vi "1A Interpret NMEA Sentence.vi"(11 "NMEA Sentence":string) -> ()   [LabVIEW 2011]
doc: "Interprets the NMEA 0813 sentences that we are using from our Airmar PB200 WeatherStation sensor.\nBy Jaime McCandless\nTODO: finish implementing NMEA sentences"
uses:
  2-Think/2 Typedefs/UTM Location.ctl
  2-Think/2 Typedefs/heading.ctl
  2-Think/2 Typedefs/Velocity.ctl
  2-Think/2 Typedefs/apparent wind.ctl
  2-Think/2 Typedefs/pitch and roll.ctl
  2-Think/2 Globals/2 Global.vi
  <vilib>/regexp/Match Regular Expression.xnode
panel:
  out "Defiltering Wind Data":bool=TRUE
  in  "UTC Time Zone":i32=-5
  in  "Tab Control":T1(tab)
  out "GPS (GGA) Data":T2
  out "GPS (GLL) Data":T3
  out "GPGSA Data":T4
  out "UTC Time":timestamp
  out "Local Time":timestamp
  out "Lattitude (ddmm.mmmm)":dbl format="%_8g"
  out "Lattitude North/South":string
  out "Longitude (ddmm.mmmm)":dbl format="%_8g"
  out "Longitude East/West":string
  out "Speed over ground (knots)":dbl format="%_3g"
  out "Course over ground (degrees)":dbl format="%_4g"
  out "Magnetic Variation (degrees)":dbl format="%_4g"
  out "Variation East/West":string
  out "GPS (RMC) Data":T5 {"Course over ground (degrees)" format="%#.6g"; "Speed over ground (knots)" format="%#.6g"; "Magnetic Variation (degrees)" format="%#.6g"; "Longitude (ddmm.mmmm)" format="%#.6g"; "Lattitude (ddmm.mmmm)" format="%#.6g"}
  out "GPS Data Valid?":bool
  out "Robot UTM Location":T6 {"North" format="%#_10f"; "East" format="%#_8f"}
  out "GPS (VTG) Data":T7
  out "Heading":dbl
  out "Turn (ROT) Data":T8
  out "Meteorological Data":T9
  out "Theoretical true wind direction":T10(graph)
  out "Relative wind direction":cluster{dbl, "Filtered Value Out":dbl}(graph)
  out "Wind (MWV) Data, Theoretical":T11
  out "Wind (MWV) Data, Relative":T11
  out "Transducer (XDR) B Data":cluster{"Pitch (deg)":dbl, "Roll (deg)":dbl}
  out "Transducer (XDR) A Data":T12
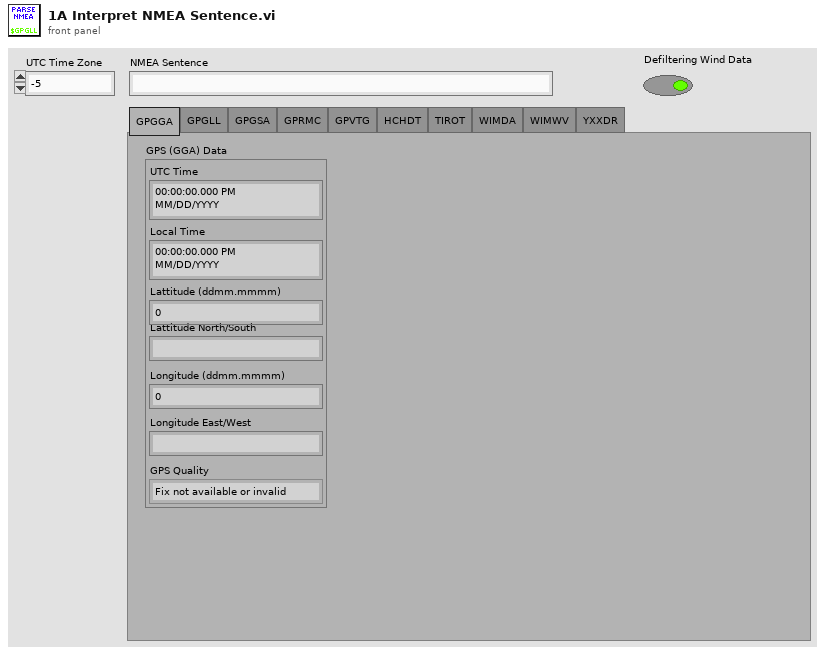
[diagram p1: front panel]
types:
  T1 = enum32{"GPGGA", "GPGLL", "GPGSA", "GPRMC", "GPVTG", "HCHDT", "TIROT", "WIMDA", "WIMWV", "YXXDR"}
  T2 = cluster{"UTC Time":timestamp, "Local Time":timestamp, "Lattitude (ddmm.mmmm)":dbl, "Lattitude North/South":string, "Longitude (ddmm.mmmm)":dbl, "Longitude East/West":string, "GPS Quality":enum16{"Fix not available or invalid", "GPS SPS Mode, fix valid", "Differential GPS, SPS Mode, fix valid", "GPS PPS Mode, fix valid", "Real Time Kinematic (RTK)", "Float RTK", "Estimated (dead reckoning) Mode", "Manual Input Mode", "Simulator Mode"}}
  T3 = cluster{"UTC Time":timestamp, "Local Time":timestamp, "Lattitude (ddmm.mmmm)":dbl, "Lattitude North/South":string, "Longitude (ddmm.mmmm)":dbl, "Longitude East/West":string, "GPS Mode":string, "GPS Data Valid?":bool}
  T4 = cluster{"Mode":string, "Fix Strength":i32, "Satellite IDs":i32[], "PDOP":dbl, "HDOP":dbl, "VDOP":dbl}
  T5 = cluster{"UTC Time":timestamp, "Local Time":timestamp, "Lattitude (ddmm.mmmm)":dbl, "Lattitude North/South":string, "Longitude (ddmm.mmmm)":dbl, "Longitude East/West":string, "Magnetic Variation (degrees)":dbl, "Variation East/West":string, "Speed over ground (knots)":dbl, "Course over ground (degrees)":dbl}
  T6 = typedef "UTM Location.ctl" = cluster{"UTM Zone":dbl, "Hemisphere":enum16{"North", "South"}, "East":dbl, "North":dbl}
  T7 = cluster{"Course Over Ground (True)":dbl, "Course Over Ground (Magnetic)":dbl, "Speed Over Ground (Knots)":dbl, "Speed Over Ground (km/hr)":dbl, "GPS Mode":string}
  T8 = cluster{"Rate of Turn (deg/min)":dbl, "Turn Rotation Data Valid?":bool}
  T9 = cluster{"Barometric Pressure (inches of mercury)":dbl, "Barometric Pressure (bars)":dbl, "Air temperature (degC)":dbl, "Relative humidity (%)":dbl, "Wind direction, True (deg)":dbl, "Wind direction, Magnetic (deg)":dbl, "Wind speed (knots)":dbl, "Wind speed (m/s)":dbl}
  T10 = cluster{"Robot\nHeading ":dbl, "Robot\nHeading ":dbl}
  T11 = cluster{"Angle relative to boat (deg)":dbl, "Wind Data Valid?":bool, "Wind speed (knots)":dbl, "True (T) or Relative (R)":string}
  T12 = cluster{"Calc. Relative Wind Chill (degC)":dbl, "Calc. Theoretical Wind Chill (degC)":dbl, "Calc. Heat Index (degC)":dbl, "Meas. Barometric Pressure (bars)":dbl}
  T13 = cluster{"second":i32, "minute":i32, "hour":i32, "day of month":i32, "month":i32, "year":i32, "day of week":i32, "day of year":i32, "is DST":i32}
  T14 = typedef "heading.ctl" = dbl
  T15 = typedef "Velocity.ctl" = cluster{"East":dbl, "North":dbl}
  T16 = typedef "apparent wind.ctl" = cluster{"Toward Fore":dbl, "Toward Starboard":dbl}
  T17 = typedef "pitch and roll.ctl" = cluster{"Pitch":dbl, "Roll":dbl}
  T18 = typedef "generalized sensor status.ctl" = cluster{"Sensor Connected":T19, "Sensor Initialized":T19, "Sensor OK":T19, "Latest Error String":string, "GPS Lock":T19}
  T19 = typedef "indicator LED.ctl" = bool
  T20 = cluster{"Robot\nHeading ":T14, "Robot\nHeading ":T14}
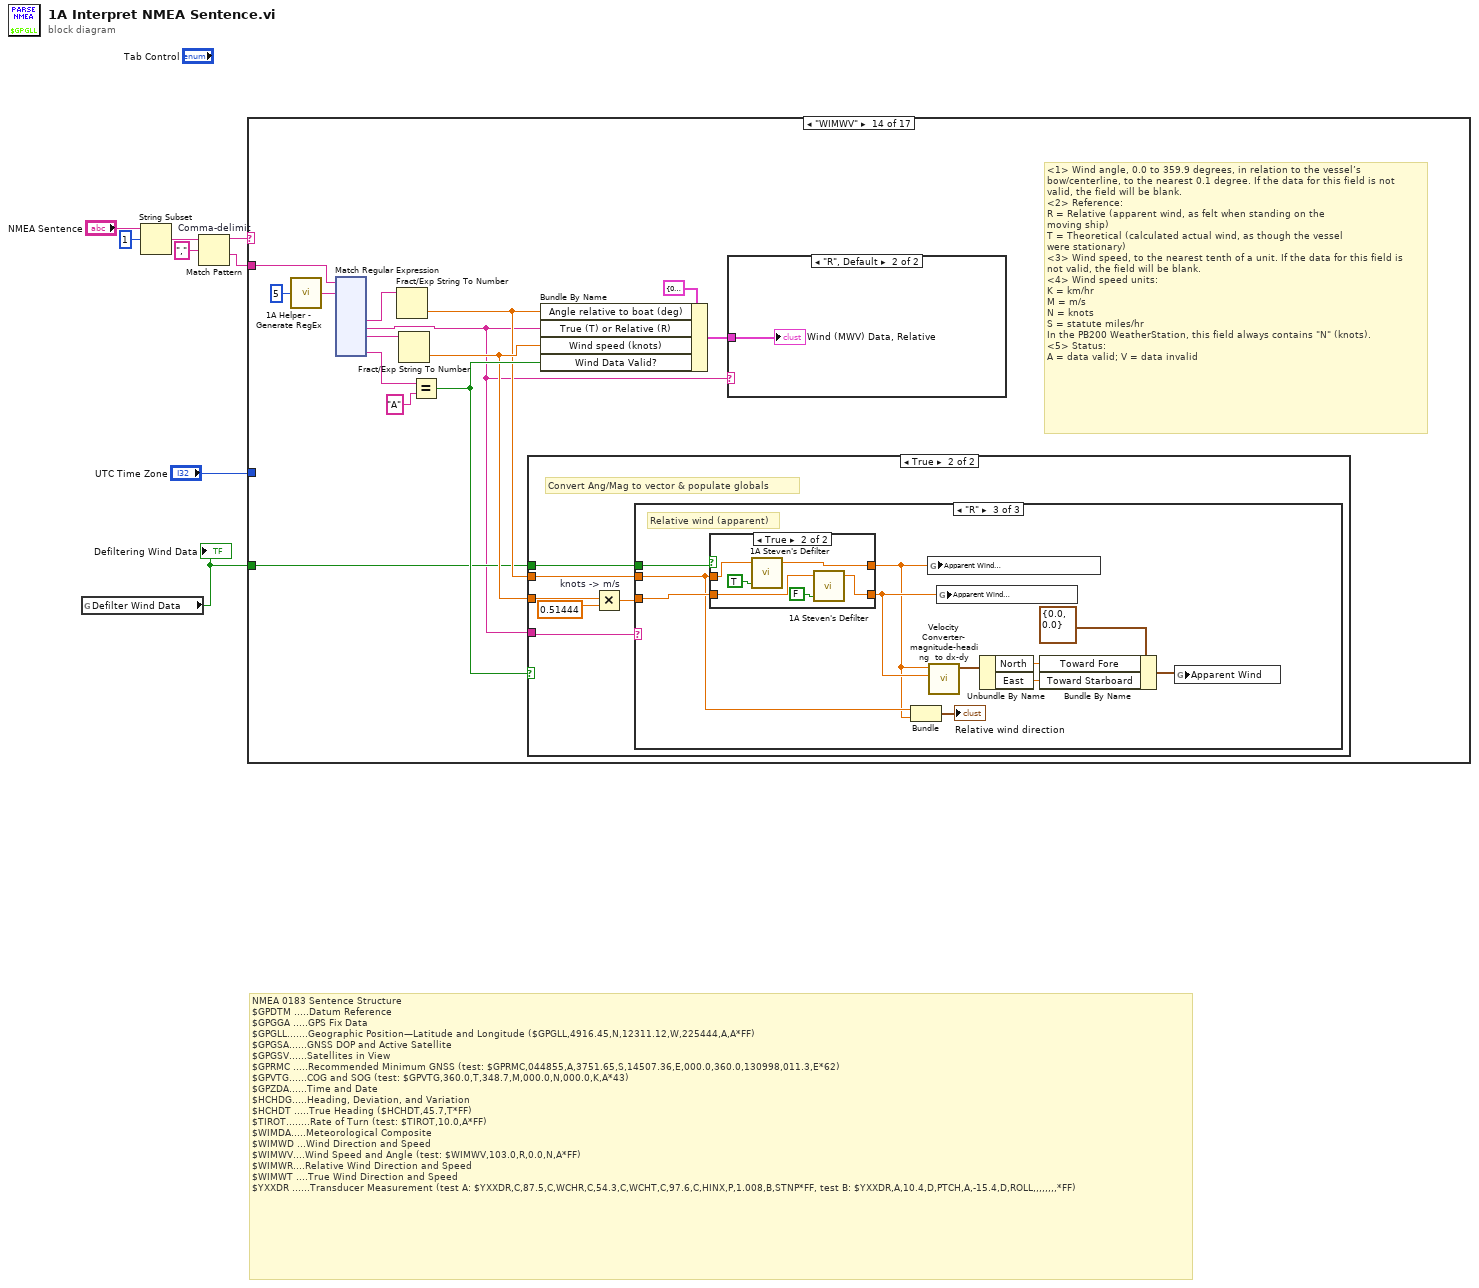
[diagram p0: block diagram]
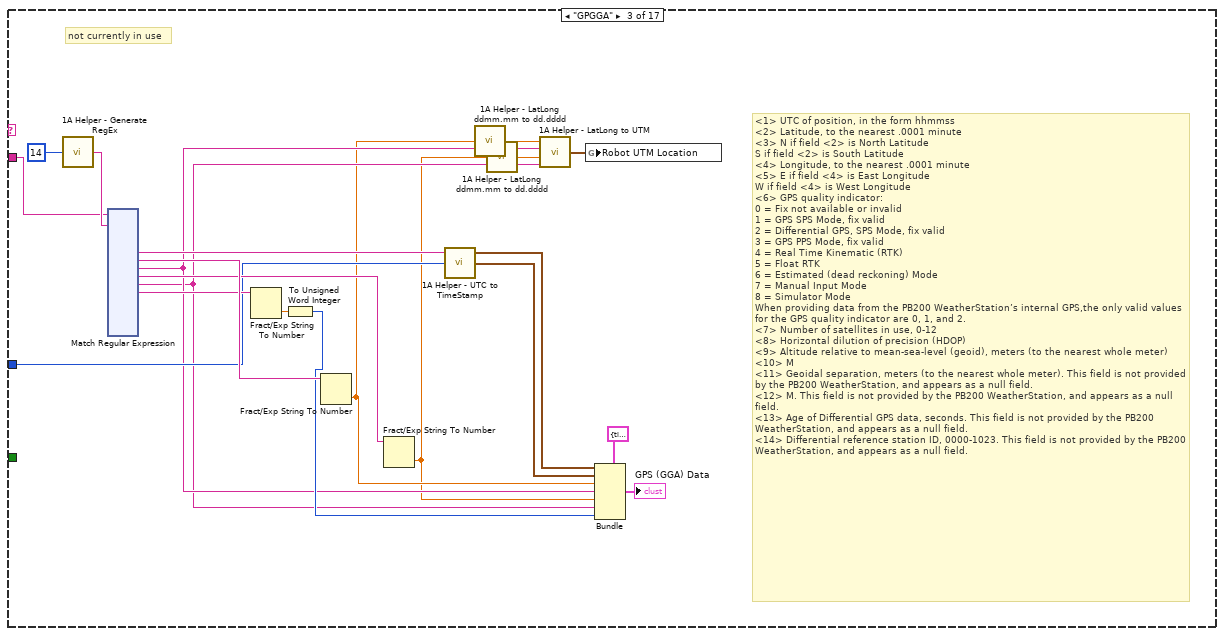
[diagram p4: hidden frame]
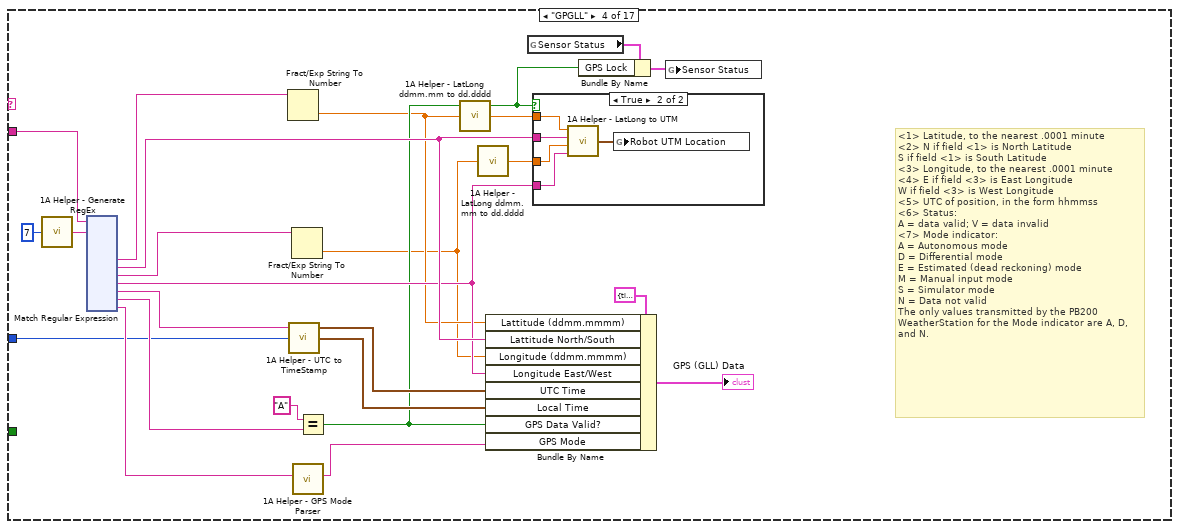
[diagram p5: hidden frame]
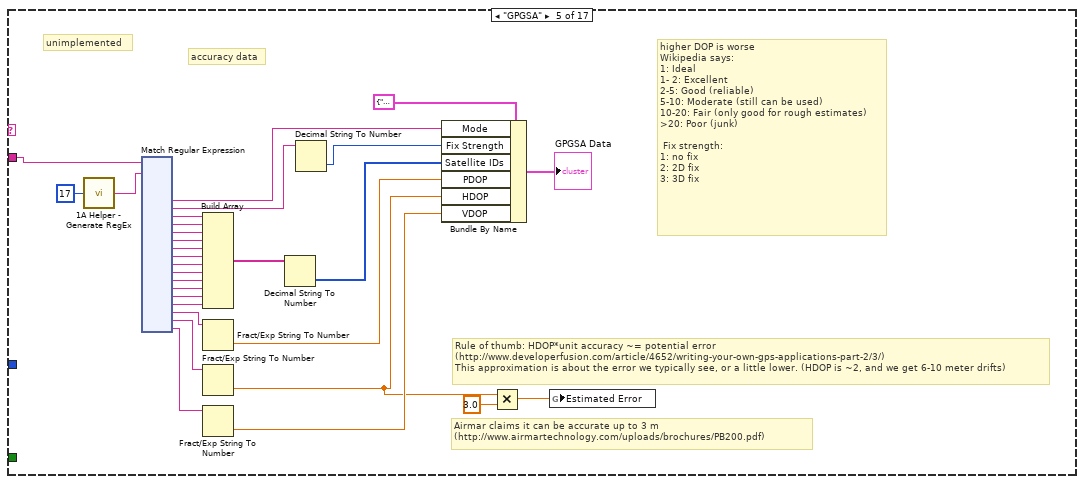
[diagram p7: hidden frame]
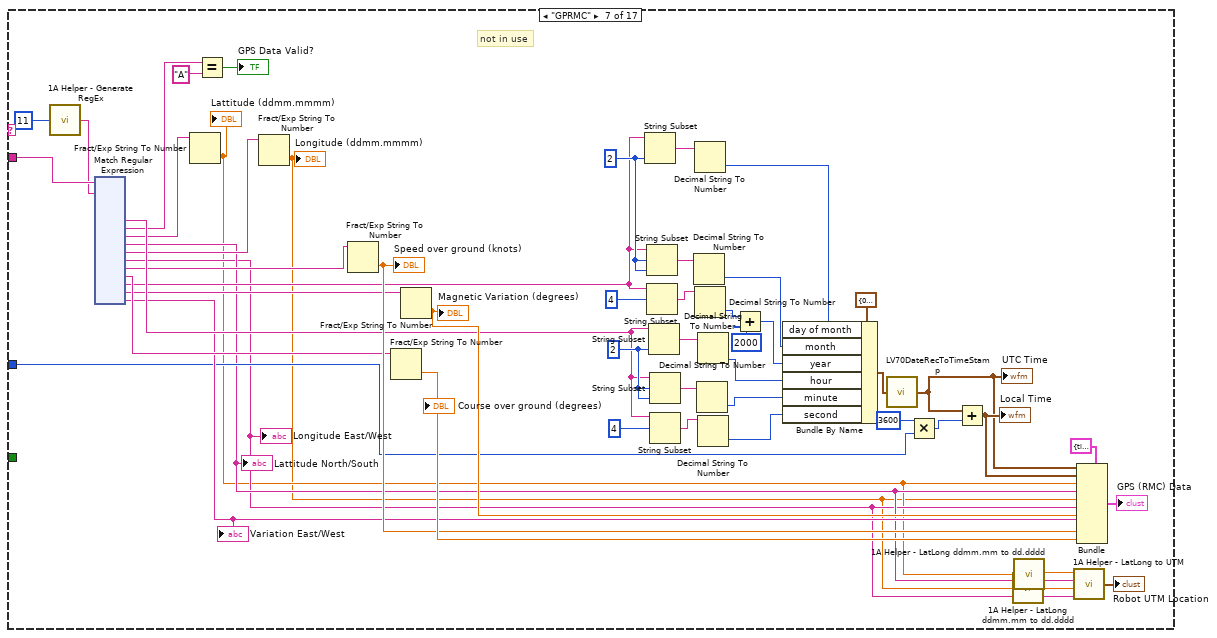
[diagram p9: hidden frame]
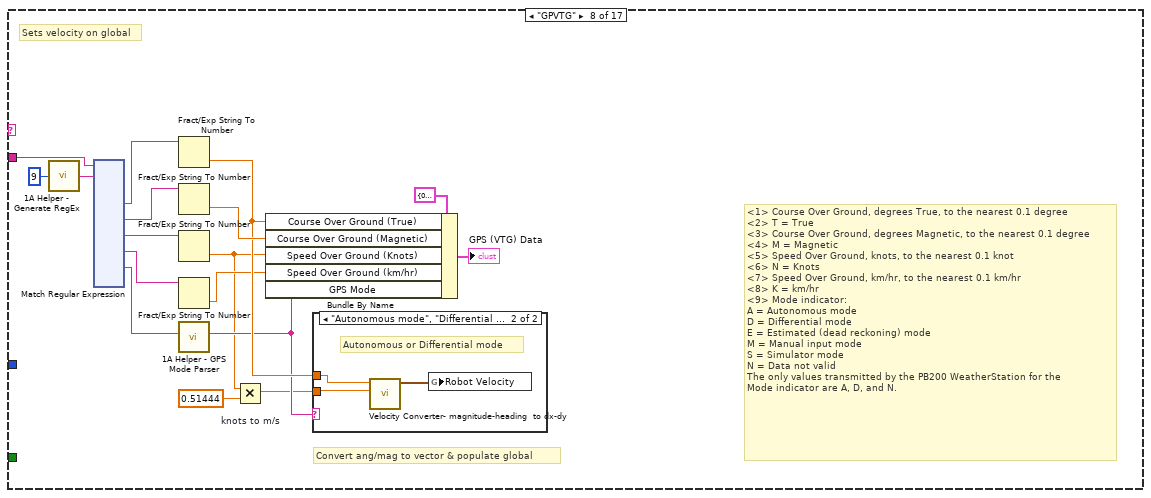
[diagram p10: hidden frame]
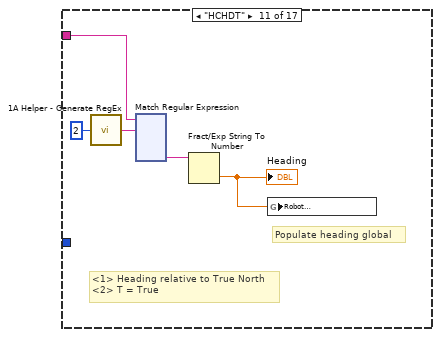
[diagram p14: hidden frame]
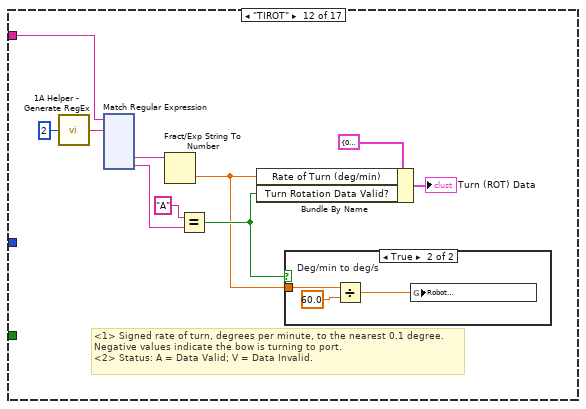
[diagram p15: hidden frame]
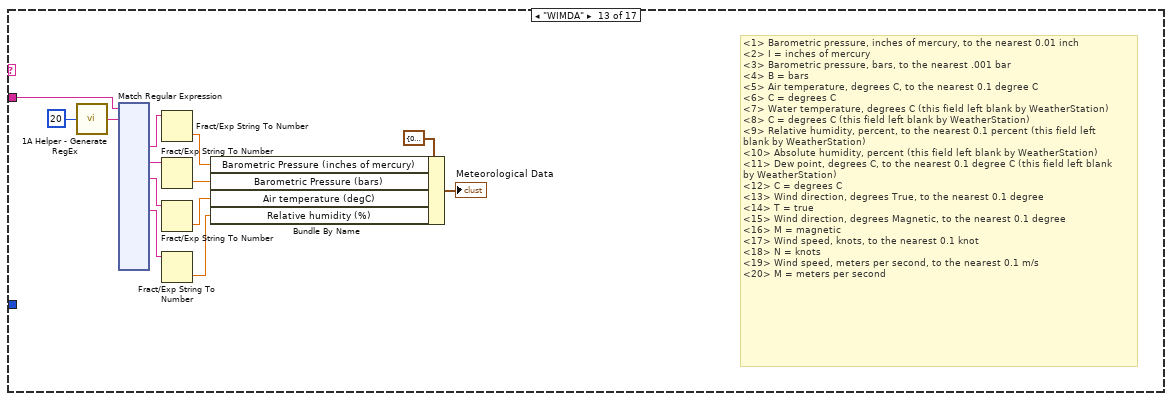
[diagram p17: hidden frame]
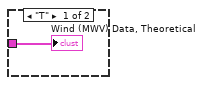
[diagram p18: hidden frame]
diagram:
  # "NMEA 0183 Sentence Structure\n$GPDTM .....Datum Reference\n$GPGGA .....GPS Fix Data\n$GPGLL.......Geographic Position—Latitude and Longitude ($GPGLL,4916.45,N,12311.12,W,225444,A,A*FF)\n$GPGSA......GNSS DOP and Active Satellite\n$GPGSV......Satellites in View\n$GPRMC .....Recommended Minimum GNSS (test: $GPRMC,044855,A,3751.65,S,14507.36,E,000.0,360.0,130998,011.3,E*62)\n$GPVTG......COG and SOG (test: $GPVTG,360.0,T,348.7,M,000.0,N,000.0,K,A*43)\n$GPZDA......Time and Date\n$HCHDG.....Heading, Deviation, and Variation\n$HCHDT .....True Heading ($HCHDT,45.7,T*FF)\n$TIROT........Rate of Turn (test: $TIROT,10.0,A*FF)\n$WIMDA.....Meteorological Composite\n$WIMWD ...Wind Direction and Speed\n$WIMWV....Wind Speed and Angle (test: $WIMWV,103.0,R,0.0,N,A*FF)\n$WIMWR....Relative Wind Direction and Speed\n$WIMWT ....True Wind Direction and Speed\n$YXXDR ......Transducer Measurement (test A: $YXXDR,C,87.5,C,WCHR,C,54.3,C,WCHT,C,97.6,C,HINX,P,1.008,B,STNP*FF, test B: $YXXDR,A,10.4,D,PTCH,A,-15.4,D,ROLL,,,,,,,,*FF)"
  n1 = global read "2 Global.vi" "Defilter Wind Data"() -> (w1:bool)
  "Defiltering Wind Data" <- w1
  n2 = String Subset(string="NMEA Sentence", offset (0)=1) -> (substring=w5:string)  [unwired: 1 in]
  n3 = Match Pattern "Comma-delimit"(string=w5, regular expression=",") -> (before substring=w6:string, after substring=w7:string)  [unwired: 1 in, 2 out]
  n4 = case shown="\"WIMWV\"" w6 {
    tunnel: w7 -> [_ _ w27 w171 w330 _ w479 w648 _ _ w779 w901 w1032 w1172 _ _ w1344]
    tunnel: "UTC Time Zone" -> [_ _ w16 w163 _ _ w467 _ _ _ _ _ _ _ _ _ _]
    tunnel: w1 -> [_ _ _ _ _ _ _ _ _ _ _ _ _ w1164 _ _ _]
    frame "", Default {
    }
    frame "GPDTM" {
      # "unimplemented"
    }
    frame "GPGGA" {
      # "not currently in use"
      # "<1> UTC of position, in the form hhmmss\n<2> Latitude, to the nearest .0001 minute\n<3> N if field <2> is North Latitude\nS if field <2> is South Latitude\n<4> Longitude, to the nearest .0001 minute\n<5> E if field <4> is East Longitude\nW if field <4> is West Longitude\n<6> GPS quality indicator:\n0 = Fix not available or invalid\n1 = GPS SPS Mode, fix valid\n2 = Differential GPS, SPS Mode, fix valid\n3 = GPS PPS Mode, fix valid\n4 = Real Time Kinematic (RTK)\n5 = Float RTK\n6 = Estimated (dead reckoning) Mode\n7 = Manual Input Mode\n8 = Simulator Mode\nWhen providing data from the PB200 WeatherStation’s internal GPS,the only valid values for the GPS quality indicator are 0, 1, and 2.\n<7> Number of satellites in use, 0-12\n<8> Horizontal dilution of precision (HDOP)\n<9> Altitude relative to mean-sea-level (geoid), meters (to the nearest whole meter)\n<10> M\n<11> Geoidal separation, meters (to the nearest whole meter). This field is not provided by the PB200 WeatherStation, and appears as a null field.\n<12> M. This field is not provided by the PB200 WeatherStation, and appears as a null field.\n<13> Age of Differential GPS data, seconds. This field is not provided by the PB200 WeatherStation, and appears as a null field.\n<14> Differential reference station ID, 0000-1023. This field is not provided by the PB200 WeatherStation, and appears as a null field."
      n5 = call "1A Helper - Generate RegEx.vi"("# Datums"=14) -> ("RegEx"=w28:string)
      n6 = xnode "Match Regular Expression"("input string"=w27, "regular expression"=w28) -> ("submatch 1"=w19:string, "submatch 2"=w25:string, "submatch 3"=w14:string, "submatch 4"=w24:string, "submatch 5"=w13:string, "submatch 6"=w23:string)  [unwired: 4 in, 10 out]
      n7 = Fract/Exp String To Number(string=w23) -> (number=w22:dbl)  [unwired: 3 in, 1 out]
      n8 = To Unsigned Word Integer(number=w22) -> (unsigned 16bit integer=w21:u16)
      n9 = Fract/Exp String To Number(string=w25) -> (number=w11:dbl)  [unwired: 3 in, 1 out]
      n10 = Fract/Exp String To Number(string=w24) -> (number=w9:dbl)  [unwired: 3 in, 1 out]
      n11 = call "1A Helper - UTC to TimeStamp.vi"("UTC Time Zone in"=w16, "UTC (hhmmss)"=w19) -> ("Local Time"=w17:timestamp, "UTC Time"=w18:timestamp)  [unwired: 2 in]
      n12 = call "1A Helper - LatLong ddmm.mm to dd.dddd.vi"("Lattitude/Longitude in ddmm.mmmm"=w11) -> ("Latitude/Longitude in dd.dddddd"=w12:dbl)
      n13 = call "1A Helper - LatLong ddmm.mm to dd.dddd.vi"("Lattitude/Longitude in ddmm.mmmm"=w9) -> ("Latitude/Longitude in dd.dddddd"=w10:dbl)
      n14 = call "1A Helper - LatLong to UTM.vi"("East/West"=w13, "Longitude"=w10, "North/South"=w14, "Latitude"=w12) -> ("Robot UTM Location"=w15:T6)
      n15 = global write "2 Global.vi" "Robot UTM Location"(w15) -> ()
      n16 = Bundle(cluster=T2 {"UTC Time"=timestamp(0 s since 1904-01-01), "Local Time"=timestamp(0 s since 1904-01-01), "Lattitude (ddmm.mmmm)"=0.0, "Lattitude North/South"="", "Longitude (ddmm.mmmm)"=0.0, "Longitude East/West"="", "GPS Quality"=enum."GPS SPS Mode, fix valid"} ("Cluster"), "UTC Time"=w18, "Local Time"=w17, "Lattitude (ddmm.mmmm)"=w11, "Lattitude North/South"=w14, "Longitude (ddmm.mmmm)"=w9, "Longitude East/West"=w13, "GPS Quality"=w21) -> (→"GPS (GGA) Data":T2)
    }
    frame "GPGLL" {
      # "<1> Latitude, to the nearest .0001 minute\n<2> N if field <1> is North Latitude\nS if field <1> is South Latitude\n<3> Longitude, to the nearest .0001 minute\n<4> E if field <3> is East Longitude\nW if field <3> is West Longitude\n<5> UTC of position, in the form hhmmss\n<6> Status:\nA = data valid; V = data invalid\n<7> Mode indicator:\nA = Autonomous mode\nD = Differential mode\nE = Estimated (dead reckoning) mode\nM = Manual input mode\nS = Simulator mode\nN = Data not valid\nThe only values transmitted by the PB200 WeatherStation for the Mode indicator are A, D, and N."
      n17 = call "1A Helper - Generate RegEx.vi"("# Datums"=7) -> ("RegEx"=w175:string)
      n18 = xnode "Match Regular Expression"("input string"=w171, "regular expression"=w175) -> ("submatch 1"=w174:string, "submatch 2"=w161:string, "submatch 3"=w173:string, "submatch 4"=w160:string, "submatch 5"=w170:string, "submatch 6"=w166:string, "submatch 7"=w172:string)  [unwired: 4 in, 5 out]
      n19 = Fract/Exp String To Number(string=w174) -> (number=w156:dbl)  [unwired: 3 in, 1 out]
      n20 = call "1A Helper - UTC to TimeStamp.vi"("UTC Time Zone in"=w163, "UTC (hhmmss)"=w170) -> ("Local Time"=w165:timestamp, "UTC Time"=w164:timestamp)  [unwired: 2 in]
      n21 = Fract/Exp String To Number(string=w173) -> (number=w154:dbl)  [unwired: 3 in, 1 out]
      n22 = call "1A Helper - GPS Mode Parser.vi"("GPS Mode (Char)"=w172) -> ("GPS Mode (Description)"=w168:string)  [unwired: 6 in]
      n23 = Equal?(x="A" ("y"), y=w166) -> (x = y?=w157:bool)
      n24 = call "1A Helper - LatLong ddmm.mm to dd.dddd.vi"("Lattitude/Longitude in ddmm.mmmm"=w156) -> ("Latitude/Longitude in dd.dddddd"=w155:dbl)
      n25 = call "1A Helper - LatLong ddmm.mm to dd.dddd.vi"("Lattitude/Longitude in ddmm.mmmm"=w154) -> ("Latitude/Longitude in dd.dddddd"=w153:dbl)
      n26 = Bundle By Name(cluster=T3 {"UTC Time"=timestamp(0 s since 1904-01-01), "Local Time"=timestamp(0 s since 1904-01-01), "Lattitude (ddmm.mmmm)"=0.0, "Lattitude North/South"="", "Longitude (ddmm.mmmm)"=0.0, "Longitude East/West"="", "GPS Mode"="", "GPS Data Valid?"=FALSE} ("Cluster"), "Lattitude (ddmm.mmmm)"=w156, "Lattitude North/South"=w161, "Longitude (ddmm.mmmm)"=w154, "Longitude East/West"=w160, "UTC Time"=w164, "Local Time"=w165, "GPS Data Valid?"=w157, "GPS Mode"=w168) -> (→"GPS (GLL) Data":T3)
      n27 = global read "2 Global.vi" "Sensor Status"() -> (w158:T18)
      n28 = case shown="True" w157 {
        tunnel: w155 -> [_ w181]
        tunnel: w161 -> [_ w180]
        tunnel: w153 -> [_ w179]
        tunnel: w160 -> [_ w178]
        frame False {
        }
        frame True {
          n29 = call "1A Helper - LatLong to UTM.vi"("East/West"=w178, "Longitude"=w179, "North/South"=w180, "Latitude"=w181) -> ("Robot UTM Location"=w177:T6)
          n30 = global write "2 Global.vi" "Robot UTM Location"(w177) -> ()
        }
      }
      n31 = Bundle By Name(cluster=w158, "GPS Lock"=w157) -> (w159:T18)
      n32 = global write "2 Global.vi" "Sensor Status"(w159) -> ()
    }
    frame "GPGSA" {
      # "Airmar claims it can be accurate up to 3 m\n(http://www.airmartechnology.com/uploads/brochures/PB200.pdf)"
      # "Rule of thumb: HDOP*unit accuracy ~= potential error\n(http://www.developerfusion.com/article/4652/writing-your-own-gps-applications-part-2/3/)\nThis approximation is about the error we typically see, or a little lower. (HDOP is ~2, and we get 6-10 meter drifts)"
      # "higher DOP is worse\nWikipedia says:\n1: Ideal\n1- 2: Excellent\n2-5: Good (reliable)\n5-10: Moderate (still can be used)\n10-20: Fair (only good for rough estimates)\n>20: Poor (junk)\n\n Fix strength: \n1: no fix\n2: 2D fix\n3: 3D fix"
      # "accuracy data"
      # "unimplemented"
      n33 = call "1A Helper - Generate RegEx.vi"("# Datums"=17) -> ("RegEx"=w329:string)
      n34 = xnode "Match Regular Expression"("input string"=w330, "regular expression"=w329) -> ("submatch 1"=w326:string, "submatch 2"=w325:string, "submatch 3"=w323:string, "submatch 4"=w322:string, "submatch 5"=w321:string, "submatch 6"=w320:string, "submatch 7"=w319:string, "submatch 8"=w318:string, "submatch 9"=w317:string, "submatch 10"=w316:string, "submatch 11"=w315:string, "submatch 12"=w314:string, "submatch 13"=w313:string, "submatch 14"=w312:string, "submatch 15"=w309:string, "submatch 16"=w307:string, "submatch 17"=w306:string)  [unwired: 4 in, 5 out]
      n35 = Build Array(w323, w322, w321, w320, w319, w318, w317, w316, w315, w314, w313, w312) -> (w311:string[])
      n36 = Fract/Exp String To Number(string=w309) -> (number=w308:dbl)  [unwired: 3 in, 1 out]
      n37 = Fract/Exp String To Number(string=w307) -> (number=w303:dbl)  [unwired: 3 in, 1 out]
      n38 = Fract/Exp String To Number(string=w306) -> (number=w305:dbl)  [unwired: 3 in, 1 out]
      n39 = Decimal String To Number(string=w311) -> (number=w310:i32[])  [unwired: 2 in, 1 out]
      n40 = Decimal String To Number(string=w325) -> (number=w324:i32)  [unwired: 2 in, 1 out]
      n41 = Bundle By Name(cluster=T4 {"Mode"="", "Fix Strength"=0, "Satellite IDs"=[], "PDOP"=0.0, "HDOP"=0.0, "VDOP"=0.0} ("GPGSA Data"), "Mode"=w326, "Fix Strength"=w324, "Satellite IDs"=w310, "PDOP"=w308, "HDOP"=w303, "VDOP"=w305) -> (→"GPGSA Data":T4)
      n42 = Multiply(x=w303, y=3.0) -> (x*y=w301:dbl)
      n43 = global write "2 Global.vi" "Estimated Error"(w301) -> ()
    }
    frame "GPGSV" {
      # "unimplemented"
    }
    frame "GPRMC" {
      w497 = 2 ("length (rest)")
      w487 = 2 ("length (rest)")
      # "not in use"
      n44 = call "1A Helper - Generate RegEx.vi"("# Datums"=11) -> ("RegEx"=w469:string)
      n45 = xnode "Match Regular Expression"("input string"=w479, "regular expression"=w469) -> ("submatch 1"=w478:string, "submatch 2"=w477:string, "submatch 3"=w476:string, "submatch 4"=w466:string, "submatch 5"=w475:string, "submatch 6"=w465:string, "submatch 7"=w474:string, "submatch 8"=w473:string, "submatch 9"=w472:string, "submatch 10"=w471:string, "submatch 11"=w470:string)  [unwired: 4 in, 5 out]
      "Lattitude North/South" <- w466
      "Longitude East/West" <- w465
      "Variation East/West" <- w470
      n46 = Fract/Exp String To Number(string=w476) -> (number=w462:dbl)  [unwired: 3 in, 1 out]
      "Lattitude (ddmm.mmmm)" <- w462
      n47 = Equal?(x=w477, y="A") -> (x = y?=→"GPS Data Valid?":bool)
      n48 = Fract/Exp String To Number(string=w475) -> (number=w460:dbl)  [unwired: 3 in, 1 out]
      "Longitude (ddmm.mmmm)" <- w460
      n49 = Fract/Exp String To Number(string=w474) -> (number=w507:dbl)  [unwired: 3 in, 1 out]
      "Speed over ground (knots)" <- w507
      n50 = Fract/Exp String To Number(string=w473) -> (number=w508:dbl)  [unwired: 3 in, 1 out]
      "Course over ground (degrees)" <- w508
      n51 = Fract/Exp String To Number(string=w471) -> (number=w506:dbl)  [unwired: 3 in, 1 out]
      "Magnetic Variation (degrees)" <- w506
      n52 = String Subset(string=w472, length (rest)=w497) -> (substring=w498:string)  [unwired: 1 in]
      n53 = String Subset(string=w472, offset (0)=w497, length (rest)=w497) -> (substring=w496:string)
      n54 = String Subset(string=w472, offset (0)=4) -> (substring=w494:string)  [unwired: 1 in]
      n55 = String Subset(string=w478, length (rest)=w487) -> (substring=w483:string)  [unwired: 1 in]
      n56 = String Subset(string=w478, offset (0)=w487, length (rest)=w487) -> (substring=w489:string)
      n57 = String Subset(string=w478, offset (0)=4) -> (substring=w491:string)  [unwired: 1 in]
      n58 = Decimal String To Number(string=w496) -> (number=w500:i32)  [unwired: 2 in, 1 out]
      n59 = Decimal String To Number(string=w498) -> (number=w499:i32)  [unwired: 2 in, 1 out]
      n60 = Decimal String To Number(string=w494) -> (number=w501:i32)  [unwired: 2 in, 1 out]
      n61 = Decimal String To Number(string=w489) -> (number=w488:i32)  [unwired: 2 in, 1 out]
      n62 = Decimal String To Number(string=w483) -> (number=w486:i32)  [unwired: 2 in, 1 out]
      n63 = Decimal String To Number(string=w491) -> (number=w492:i32)  [unwired: 2 in, 1 out]
      n64 = Add(x=w501, y=2000) -> (x+y=w503:i32)
      n65 = Bundle By Name(cluster=T13 {"second"=0, "minute"=0, "hour"=0, "day of month"=0, "month"=0, "year"=0, "day of week"=0, "day of year"=0, "is DST"=0} ("date time rec"), "day of month"=w499, "month"=w500, "year"=w503, "hour"=w486, "minute"=w488, "second"=w492) -> (w484:T13)
      n66 = call <vilib>:"LV70DateRecToTimeStamp.vi"("date time rec"=w484) -> ("Time Stamp"=w504:timestamp)
      "UTC Time" <- w504
      n67 = Multiply(x=3600 ("number"), y=w467) -> (x*y=w468:i32)
      n68 = Add(x=w504, y=w468) -> (x+y=w505:timestamp)
      "Local Time" <- w505
      n69 = call "1A Helper - LatLong ddmm.mm to dd.dddd.vi"("Lattitude/Longitude in ddmm.mmmm"=w460) -> ("Latitude/Longitude in dd.dddddd"=w461:dbl)
      n70 = call "1A Helper - LatLong ddmm.mm to dd.dddd.vi"("Lattitude/Longitude in ddmm.mmmm"=w462) -> ("Latitude/Longitude in dd.dddddd"=w463:dbl)
      n71 = call "1A Helper - LatLong to UTM.vi"("East/West"=w465, "Longitude"=w461, "North/South"=w466, "Latitude"=w463) -> ("Robot UTM Location"=→"Robot UTM Location":T6)
      n72 = Bundle(cluster=T5 {"UTC Time"=timestamp(0 s since 1904-01-01), "Local Time"=timestamp(0 s since 1904-01-01), "Lattitude (ddmm.mmmm)"=0.0, "Lattitude North/South"="", "Longitude (ddmm.mmmm)"=0.0, "Longitude East/West"="", "Magnetic Variation (degrees)"=0.0, "Variation East/West"="", "Speed over ground (knots)"=0.0, "Course over ground (degrees)"=0.0} ("Cluster"), "UTC Time"=w504, "Local Time"=w505, "Lattitude (ddmm.mmmm)"=w462, "Lattitude North/South"=w466, "Longitude (ddmm.mmmm)"=w460, "Longitude East/West"=w465, "Magnetic Variation (degrees)"=w506, "Variation East/West"=w470, "Speed over ground (knots)"=w507, "Course over ground (degrees)"=w508) -> (→"GPS (RMC) Data":T5)
    }
    frame "GPVTG" {
      # "Convert ang/mag to vector & populate global"
      # "Sets velocity on global"
      # "<1> Course Over Ground, degrees True, to the nearest 0.1 degree\n<2> T = True\n<3> Course Over Ground, degrees Magnetic, to the nearest 0.1 degree\n<4> M = Magnetic\n<5> Speed Over Ground, knots, to the nearest 0.1 knot\n<6> N = Knots\n<7> Speed Over Ground, km/hr, to the nearest 0.1 km/hr\n<8> K = km/hr\n<9> Mode indicator:\nA = Autonomous mode\nD = Differential mode\nE = Estimated (dead reckoning) mode\nM = Manual input mode\nS = Simulator mode\nN = Data not valid\nThe only values transmitted by the PB200 WeatherStation for the\nMode indicator are A, D, and N."
      n73 = call "1A Helper - Generate RegEx.vi"("# Datums"=9) -> ("RegEx"=w649:string)
      n74 = xnode "Match Regular Expression"("input string"=w648, "regular expression"=w649) -> ("submatch 1"=w645:string, "submatch 3"=w644:string, "submatch 5"=w642:string, "submatch 7"=w641:string, "submatch 9"=w640:string)  [unwired: 4 in, 11 out]
      n75 = Fract/Exp String To Number(string=w645) -> (number=w639:dbl)  [unwired: 3 in, 1 out]
      n76 = Fract/Exp String To Number(string=w644) -> (number=w643:dbl)  [unwired: 3 in, 1 out]
      n77 = Fract/Exp String To Number(string=w642) -> (number=w636:dbl)  [unwired: 3 in, 1 out]
      n78 = Fract/Exp String To Number(string=w641) -> (number=w638:dbl)  [unwired: 3 in, 1 out]
      n79 = call "1A Helper - GPS Mode Parser.vi"("GPS Mode (Char)"=w640) -> ("GPS Mode (Description)"=w637:string)  [unwired: 6 in]
      n80 = Multiply "knots to m/s"(x=w636, y=0.51444) -> (x*y=w635:dbl)
      n81 = Bundle By Name(cluster=T7 {"Course Over Ground (True)"=0.0, "Course Over Ground (Magnetic)"=0.0, "Speed Over Ground (Knots)"=0.0, "Speed Over Ground (km/hr)"=0.0, "GPS Mode"=""} ("GPS (VTG) Data 2"), "Course Over Ground (True)"=w639, "Course Over Ground (Magnetic)"=w643, "Speed Over Ground (Knots)"=w636, "Speed Over Ground (km/hr)"=w638, "GPS Mode"=w637) -> (→"GPS (VTG) Data":T7)
      n82 = case shown="\"Autonomous mode\", \"Differential mode\"" w637 {
        tunnel: w639 -> [_ w653]
        tunnel: w635 -> [_ w652]
        frame "Data not valid", Default {
          # "Data not valid"
        }
        frame "Autonomous mode", "Differential mode" {
          # "Autonomous or Differential mode"
          n83 = call "Velocity Converter- magnitude-heading  to dx-dy.vi"("Magnitude"=w652, "Heading"=w653) -> ("Vector Out"=w651:T15)  [unwired: 9 in]
          n84 = global write "2 Global.vi" "Robot Velocity"(w651) -> ()
        }
      }
    }
    frame "GPZDA" {
      # "<1> UTC time of day, in the form hhmmss\n<2> UTC day, 01 to 31\n<3> UTC month, 01 to 12\n<4> UTC year (four digits, e.g. 2006)\n<5> Local time zone hours, 00 to +/-13 hrs\n<6> Local time zone minutes, 00 to +59"
    }
    frame "HCHDG " {
      # "<1> Magnetic sensor heading, degrees, to the nearest 0.1 degree.\n<2> Magnetic deviation, degrees east or west, to the nearest 0.1 degree.\n<3> E if field <2> is degrees East\nW if field <2> is degrees West\n<4> Magnetic variation, degrees east or west, to the nearest 0.1 degree.\n<5> E if field <4> is degrees East\nW if field <4> is degrees West"
    }
    frame "HCHDT" {
      # "Populate heading global"
      # "<1> Heading relative to True North\n<2> T = True"
      n85 = call "1A Helper - Generate RegEx.vi"("# Datums"=2) -> ("RegEx"=w780:string)
      n86 = xnode "Match Regular Expression"("input string"=w779, "regular expression"=w780) -> ("submatch 1"=w778:string)  [unwired: 4 in, 5 out]
      n87 = Fract/Exp String To Number(string=w778) -> (number=w777:dbl)  [unwired: 3 in, 1 out]
      "Heading" <- w777
      n88 = global write "2 Global.vi" "Robot\nHeading"(w777) -> ()
    }
    frame "TIROT" {
      # "<1> Signed rate of turn, degrees per minute, to the nearest 0.1 degree.\nNegative values indicate the bow is turning to port.\n<2> Status: A = Data Valid; V = Data Invalid."
      n89 = call "1A Helper - Generate RegEx.vi"("# Datums"=2) -> ("RegEx"=w903:string)
      n90 = xnode "Match Regular Expression"("input string"=w901, "regular expression"=w903) -> ("submatch 1"=w902:string, "submatch 2"=w897:string)  [unwired: 4 in, 5 out]
      n91 = Fract/Exp String To Number(string=w902) -> (number=w895:dbl)  [unwired: 3 in, 1 out]
      n92 = Equal?(x="A" ("y"), y=w897) -> (x = y?=w896:bool)
      n93 = Bundle By Name(cluster=T8 {"Rate of Turn (deg/min)"=0.0, "Turn Rotation Data Valid?"=TRUE} ("Turn (ROT) Data 2"), "Rate of Turn (deg/min)"=w895, "Turn Rotation Data Valid?"=w896) -> (→"Turn (ROT) Data":T8)
      n94 = case shown="True" w896 {
        tunnel: w895 -> [_ w906]
        frame False {
        }
        frame True {
          n95 = Divide "Deg/min to deg/s"(x=w906, y=60.0) -> (x/y=w907:dbl)
          n96 = global write "2 Global.vi" "Robot\nRate of Turn"(w907) -> ()
        }
      }
    }
    frame "WIMDA" {
      # "<1> Barometric pressure, inches of mercury, to the nearest 0.01 inch\n<2> I = inches of mercury\n<3> Barometric pressure, bars, to the nearest .001 bar\n<4> B = bars\n<5> Air temperature, degrees C, to the nearest 0.1 degree C\n<6> C = degrees C\n<7> Water temperature, degrees C (this field left blank by WeatherStation)\n<8> C = degrees C (this field left blank by WeatherStation)\n<9> Relative humidity, percent, to the nearest 0.1 percent (this field left\nblank by WeatherStation)\n<10> Absolute humidity, percent (this field left blank by WeatherStation)\n<11> Dew point, degrees C, to the nearest 0.1 degree C (this field left blank\nby WeatherStation)\n<12> C = degrees C\n<13> Wind direction, degrees True, to the nearest 0.1 degree\n<14> T = true\n<15> Wind direction, degrees Magnetic, to the nearest 0.1 degree\n<16> M = magnetic\n<17> Wind speed, knots, to the nearest 0.1 knot\n<18> N = knots\n<19> Wind speed, meters per second, to the nearest 0.1 m/s\n<20> M = meters per second"
      n97 = call "1A Helper - Generate RegEx.vi"("# Datums"=20) -> ("RegEx"=w1033:string)
      n98 = xnode "Match Regular Expression"("input string"=w1032, "regular expression"=w1033) -> ("submatch 1"=w1026:string, "submatch 3"=w1025:string, "submatch 5"=w1024:string, "submatch 9"=w1023:string)  [unwired: 4 in, 17 out]
      n99 = Fract/Exp String To Number(string=w1026) -> (number=w1030:dbl)  [unwired: 3 in, 1 out]
      n100 = Fract/Exp String To Number(string=w1025) -> (number=w1029:dbl)  [unwired: 3 in, 1 out]
      n101 = Fract/Exp String To Number(string=w1024) -> (number=w1028:dbl)  [unwired: 3 in, 1 out]
      n102 = Fract/Exp String To Number(string=w1023) -> (number=w1027:dbl)  [unwired: 3 in, 1 out]
      n103 = Bundle By Name(cluster=T9 {"Barometric Pressure (inches of mercury)"=0.0, "Barometric Pressure (bars)"=0.0, "Air temperature (degC)"=0.0, "Relative humidity (%)"=0.0, "Wind direction, True (deg)"=0.0, "Wind direction, Magnetic (deg)"=0.0, "Wind speed (knots)"=0.0, "Wind speed (m/s)"=0.0} ("Meteorological Data"), "Barometric Pressure (inches of mercury)"=w1030, "Barometric Pressure (bars)"=w1029, "Air temperature (degC)"=w1028, "Relative humidity (%)"=w1027) -> (→"Meteorological Data":T9)
    }
    frame "WIMWV" {
      # "<1> Wind angle, 0.0 to 359.9 degrees, in relation to the vessel’s\nbow/centerline, to the nearest 0.1 degree. If the data for this field is not\nvalid, the field will be blank.\n<2> Reference:\nR = Relative (apparent wind, as felt when standing on the\nmoving ship)\nT = Theoretical (calculated actual wind, as though the vessel\nwere stationary)\n<3> Wind speed, to the nearest tenth of a unit. If the data for this field is\nnot valid, the field will be blank.\n<4> Wind speed units:\nK = km/hr\nM = m/s\nN = knots\nS = statute miles/hr\nIn the PB200 WeatherStation, this field always contains \"N\" (knots).\n<5> Status:\nA = data valid; V = data invalid"
      n104 = call "1A Helper - Generate RegEx.vi"("# Datums"=5) -> ("RegEx"=w1175:string)
      n105 = xnode "Match Regular Expression"("input string"=w1172, "regular expression"=w1175) -> ("submatch 1"=w1174:string, "submatch 2"=w1163:string, "submatch 3"=w1169:string, "submatch 5"=w1168:string)  [unwired: 4 in, 6 out]
      n106 = Fract/Exp String To Number(string=w1174) -> (number=w1165:dbl)  [unwired: 3 in, 1 out]
      n107 = Fract/Exp String To Number(string=w1169) -> (number=w1166:dbl)  [unwired: 3 in, 1 out]
      n108 = Equal?(x=w1168, y="A") -> (x = y?=w1167:bool)
      n109 = case shown="True" w1167 {
        tunnel: w1166 -> [_ w1181]
        tunnel: w1165 -> [_ w1184]
        tunnel: w1163 -> [_ w1183]
        tunnel: w1164 -> [_ w1179]
        frame False {
        }
        frame True {
          # "Convert Ang/Mag to vector & populate globals"
          n110 = Multiply "knots -> m/s"(x=w1181, y=0.51444) -> (x*y=w1182:dbl)
          n111 = case shown="\"R\"" w1183 {
            tunnel: w1182 -> [_ w1189 w1213]
            tunnel: w1184 -> [_ w1193 w1209]
            tunnel: w1179 -> [_ w1190 w1212]
            frame "", Default {
            }
            frame "T" {
              # "Theoretical wind (absolute)"
              n112 = global read "2 Global.vi" "Robot\nHeading"() -> (w1194:T14)
              n113 = Add "Get relative to compass, not boat"(x=w1194, y=w1193) -> (x+y=w1192:T14)
              n114 = Quotient & Remainder(x=w1192, y=T14 360.0) -> (x-y*floor(x/y)=w1186:T14)  [unwired: 1 out]
              n115 = case shown="True" w1190 {
                tunnel: [w1200 w1207] -> w1188
                tunnel: w1189 -> [w1200 w1206]
                tunnel: w1186 -> [w1201 w1205]
                tunnel: [w1201 w1204] -> w1187
                frame False {
                }
                frame True {
                  n116 = call "1A Steven's Defilter.vi"("Angle?(F)"=FALSE, "Value In"=w1206) -> ("Filtered Value Out"=w1207:dbl)  [unwired: 3 in]
                  n117 = call "1A Steven's Defilter.vi"("Angle?(F)"=TRUE, "Value In"=w1205) -> ("Filtered Value Out"=w1204:dbl)  [unwired: 3 in]
                }
              }
              n118 = call "Velocity Converter- magnitude-heading  to dx-dy.vi"("Magnitude"=w1188, "Heading"=w1187) -> ("Vector Out"=w1199:T15)  [unwired: 9 in]
              n119 = Bundle("Robot\nHeading"=w1186, "Robot\nHeading"=w1187) -> (→"Theoretical true wind direction":T20)  [unwired: 1 in]
              n120 = global write "2 Global.vi" "Absolute Wind\nDirection (º)"(w1187) -> ()
              n121 = global write "2 Global.vi" "Absolute Wind\nSpeed"(w1188) -> ()
              n122 = Unbundle By Name(w1199) -> ("North"=w1197:dbl, "East"=w1196:dbl)
              n123 = Bundle By Name(cluster=T15 {"East"=0.0, "North"=0.0} ("Absolute Wind"), "North"=w1197, "East"=w1196) -> (w1198:T15)
              n124 = global write "2 Global.vi" "Absolute Wind"(w1198) -> ()
            }
            frame "R" {
              # "Relative wind (apparent)"
              n125 = case shown="True" w1212 {
                tunnel: [w1219 w1224] -> w1211
                tunnel: [w1220 w1223] -> w1208
                tunnel: w1209 -> [w1220 w1222]
                tunnel: w1213 -> [w1219 w1221]
                frame False {
                }
                frame True {
                  n126 = call "1A Steven's Defilter.vi"("Angle?(F)"=TRUE, "Value In"=w1222) -> ("Filtered Value Out"=w1223:dbl)  [unwired: 3 in]
                  n127 = call "1A Steven's Defilter.vi"("Angle?(F)"=FALSE, "Value In"=w1221) -> ("Filtered Value Out"=w1224:dbl)  [unwired: 3 in]
                }
              }
              n128 = Bundle(w1209, "Filtered Value Out"=w1208) -> (→"Relative wind direction":cluster{dbl, "Filtered Value Out":dbl})  [unwired: 1 in]
              n129 = global write "2 Global.vi" "Apparent Wind\nDirection (º)"(w1208) -> ()
              n130 = call "Velocity Converter- magnitude-heading  to dx-dy.vi"("Magnitude"=w1211, "Heading"=w1208) -> ("Vector Out"=w1214:T15)  [unwired: 9 in]
              n131 = global write "2 Global.vi" "Apparent Wind\nSpeed"(w1211) -> ()
              n132 = Unbundle By Name(w1214) -> ("North"=w1217:dbl, "East"=w1218:dbl)
              n133 = Bundle By Name(cluster=T16 {"Toward Fore"=0.0, "Toward Starboard"=0.0} ("Apparent Wind"), "Toward Fore"=w1217, "Toward Starboard"=w1218) -> (w1216:T16)
              n134 = global write "2 Global.vi" "Apparent Wind"(w1216) -> ()
            }
          }
        }
      }
      n135 = Bundle By Name(cluster=T11 {"Angle relative to boat (deg)"=0.0, "Wind Data Valid?"=TRUE, "Wind speed (knots)"=0.0, "True (T) or Relative (R)"=""} ("Wind (MWV) Data 2"), "Angle relative to boat (deg)"=w1165, "True (T) or Relative (R)"=w1163, "Wind speed (knots)"=w1166, "Wind Data Valid?"=w1167) -> (w1171:T11)
      n136 = case shown="\"R\", Default" w1163 {
        tunnel: w1171 -> [w1177 w1178]
        frame "T" {
          "Wind (MWV) Data, Theoretical" <- w1177
        }
        frame "R", Default {
          "Wind (MWV) Data, Relative" <- w1178
        }
      }
    }
    frame "WIMWR" {
    }
    frame "WIMWT" {
    }
    frame "YXXDR" {
      n137 = String Subset(string=w1344, length (rest)=1 ("length (rest)")) -> (substring=w1345:string)  [unwired: 1 in]
      n138 = case shown="\"A\"" w1345 {
        tunnel: w1344 -> [_ w1347 w1486]
        frame "", Default {
        }
        frame "A" {
          # "TYPE B:\n<1> A = angular displacement\n<2> Pitch: oscillation of vessel about its latitudinal axis. Bow moving up is positive. Value reported to the nearest 0.1 degree.\n<3> D = degrees\n<4> PTCH (ID indicating pitch of vessel)\n<5> A = angular displacement\n<6> Roll: oscillation of vessel about its longitudinal axis. Roll to the starboard is positive. Value reported to the nearest 0.1 degree.\n<7> D = degrees\n<8> ROLL (ID indicating roll of vessel)\n<9> Not used\n<10> Not used\n<11> Not used\n<12> Not used\n<13> Not used\n<14> Not used\n<15> Not used\n<16> Not used"
          n139 = call "1A Helper - Generate RegEx.vi"("# Datums"=8) -> ("RegEx"=w1351:string)
          n140 = xnode "Match Regular Expression"("input string"=w1347, "regular expression"=w1351) -> ("submatch 2"=w1349:string, "submatch 6"=w1348:string)  [unwired: 4 in, 19 out]
          n141 = Fract/Exp String To Number(string=w1349) -> (number=w1353:dbl)  [unwired: 3 in, 1 out]
          n142 = Fract/Exp String To Number(string=w1348) -> (number=w1352:dbl)  [unwired: 3 in, 1 out]
          n143 = Bundle By Name(cluster=cluster{"Pitch (deg)":dbl, "Roll (deg)":dbl} {"Pitch (deg)"=103.0, "Roll (deg)"=103.0} ("Transducer (XDR) B Data 2"), "Pitch (deg)"=w1353, "Roll (deg)"=w1352) -> (→"Transducer (XDR) B Data":cluster{"Pitch (deg)":dbl, "Roll (deg)":dbl})
          n144 = Bundle By Name(cluster=T17 {"Pitch"=0.0, "Roll"=0.0} ("Robot Pitch/Roll"), "Pitch"=w1353, "Roll"=w1352) -> (w1354:T17)
          n145 = global write "2 Global.vi" "Robot Pitch/Roll"(w1354) -> ()
        }
        frame "C" {
          # "TYPE A:\n<1> C = temperature\n<2> Calculated “relative” wind chill temperature, degrees Celsius, to the nearest 0.1 degree\n<3> C = degrees C\n<4> WCHR (ID indicating relative wind chill)\n<5> C = temperature\n<6> Calculated “theoretical” wind chill temperature, degrees Celsius, to the nearest 0.1 degree\n<7> C = degrees C\n<8> WCHT (ID indicating theoretical wind chill)\n<9> C = temperature\n<10> Calculated heat index, degrees Celsius, to the nearest 0.1 degree (this field left blank by WeatherStation)\n<11> C = degrees C\n<12> HINX (ID indicating heat index)\n<13> P = pressure\n<14> Actual measured barometric pressure, or \"station pressure\", bars, to the nearest 0.001 bar\n<15> B = bars\n<16> STNP (ID indicating station pressure)"
          n146 = call "1A Helper - Generate RegEx.vi"("# Datums"=16) -> ("RegEx"=w1492:string)
          n147 = xnode "Match Regular Expression"("input string"=w1486, "regular expression"=w1492) -> ("submatch 2"=w1490:string, "submatch 6"=w1489:string, "submatch 10"=w1488:string, "submatch 14"=w1487:string)  [unwired: 4 in, 17 out]
          n148 = Fract/Exp String To Number(string=w1490) -> (number=w1496:dbl)  [unwired: 3 in, 1 out]
          n149 = Fract/Exp String To Number(string=w1489) -> (number=w1495:dbl)  [unwired: 3 in, 1 out]
          n150 = Fract/Exp String To Number(string=w1488) -> (number=w1494:dbl)  [unwired: 3 in, 1 out]
          n151 = Fract/Exp String To Number(string=w1487) -> (number=w1493:dbl)  [unwired: 3 in, 1 out]
          n152 = Bundle By Name(cluster=T12 {"Calc. Relative Wind Chill (degC)"=0.0, "Calc. Theoretical Wind Chill (degC)"=0.0, "Calc. Heat Index (degC)"=0.0, "Meas. Barometric Pressure (bars)"=0.0} ("Transducer (XDR) A Data 2"), "Calc. Relative Wind Chill (degC)"=w1496, "Calc. Theoretical Wind Chill (degC)"=w1495, "Calc. Heat Index (degC)"=w1494, "Meas. Barometric Pressure (bars)"=w1493) -> (→"Transducer (XDR) A Data":T12)
        }
      }
    }
  }
